vi "rad_GetInstalledSoftware.vi"(8 "error in (no error)":errorcluster, 11 "Target settings":T1={"Hostname"="", "Serial number"="", "Product name"="", "Product code"=0, "System status"="", "Credential type"=enum."None/Unlocked", "User added?"=FALSE, "Primary NIC"={"MAC address"="", "IP Address Request Mode"=2, "IP address"="", "Subnet mask"="", "Gateway"="", "DNS server"=""}} {"Primary NIC"."IP Address Request Mode" items=["Static"=1, "DHCP/Link-Local"=2, "Link-Local Only"=4, "DHCP Only"=8]}) -> (0 "error out":errorcluster, 3 "installedSoftware":string[](array[string]))   [LabVIEW 2023]
uses:
  Targets/TypeDefs/rad_Target Information.ctl
  Targets/TypeDefs/rad_Target Network Settings.ctl
  <vilib>/nisyscfg/Get Installed Components.vi
  <vilib>/nisyscfg/Close (System).vi
  <vilib>/nisyscfg/nisyscfg.lvlib
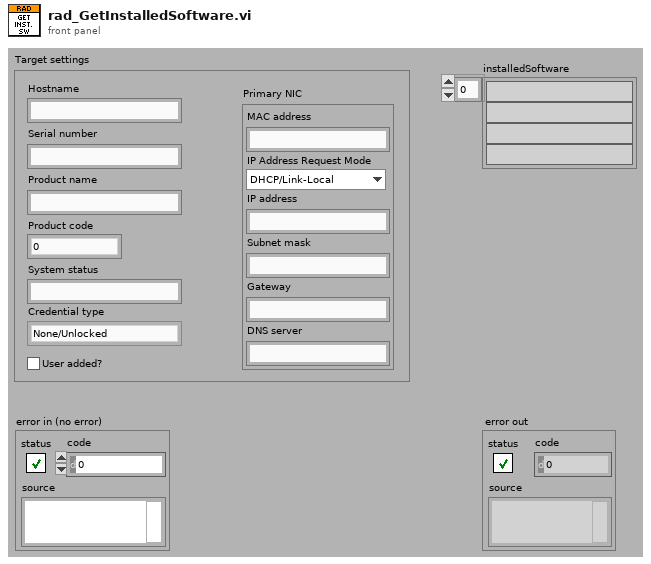
[diagram p1: front panel]
types:
  T1 = typedef "rad_Target Information.ctl" = cluster{"Hostname":string, "Serial number":string, "Product name":string, "Product code":i32, "System status":string, "Credential type":enum16{"None/Unlocked", "FTP Password", "NIAuth Credentials"}, "User added?":bool, "Primary NIC":T2}
  T2 = typedef "rad_Target Network Settings.ctl" = cluster{"MAC address":string, "IP Address Request Mode":i32, "IP address":string, "Subnet mask":string, "Gateway":string, "DNS server":string}
  T3 = typedef "nisyscfg.lvlib/Software 1.2.ctl" = cluster{"title":string, "description":string, "ID":string, "version":string, "component type":T4}
  T4 = typedef "nisyscfg.lvlib/Component Type.ctl" = u32
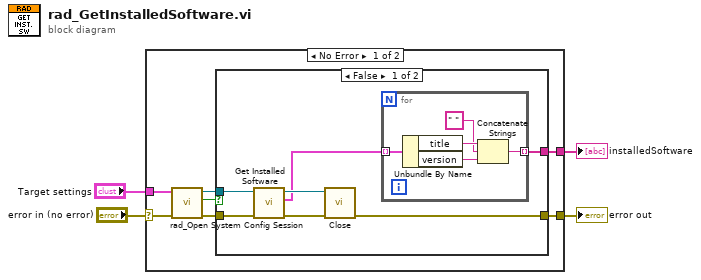
[diagram p0: block diagram]
diagram:
  n1 = case shown="No Error" "error in (no error)" {
    selector: "error in (no error)" -> [w9 w25]
    tunnel: [w11 w25] -> w4
    tunnel: [w10 _] -> w2
    tunnel: "Target settings" -> [w5 _]
    frame No Error {
      n2 = call "rad_Open System Config Session.vi"("error in (no error)"=w9, "Target settings"=w5) -> ("error out"=w7:errorcluster, "Cancelled"=w6:bool, "Session out"=w8:refnum<k21>)  [unwired: 6 in, 1 out]
      n3 = case shown="False" w6 {
        tunnel: [w16 w24] -> w11
        tunnel: [w14 _] -> w10
        tunnel: w8 -> [w13 _]
        tunnel: w7 -> [w12 w24]
        frame False {
          n4 = call-poly <vilib>:"Get Installed Software.vi"("error in (no error)"=w12, "Session in"=w13) -> ("error out"=w18:errorcluster, "Software Components"=w15:T3[], "Session out"=w17:refnum<k21>)  [unwired: 7 in]
          n5 = call-poly <vilib>:"Close.vi"("error in (no error)"=w18, "Session in"=w17) -> ("error out"=w16:errorcluster)  [unwired: 9 in]
          n6 = for {
            tunnel: w15 -> [w23] mode=indexing
            tunnel: [w19] -> w14 mode=indexing
            n7 = Unbundle By Name(w23) -> ("title"=w22:string, "version"=w21:string)
            n8 = Concatenate Strings(w22, " " ("string"), w21) -> (w19:string)
          }
        }
        frame True {
        }
      }
    }
    frame Error {
    }
  }
  "error out" <- w4
  "installedSoftware" <- w2
